vi "Read Data and Memory Array.vi"(7 "Channel (1)":i32=1, 8 "error in (no error)":errorcluster, 9 "Correction (0: Data)":u16(ring) items=["Formatted", "Corrected"], 10 "Source (0: Data)":u16(ring) items=["Data", "Memory"], 11 "VISA resource name":refnum<visa-resource-name>) -> (0 "error out":errorcluster, 1 "Secondary / Imaginary":dbl[](array[numeric]), 2 "Primary / Real":dbl[](array[numeric]), 3 "VISA resource name out":refnum<visa-resource-name>)   [LabVIEW 2011, in "Agilent ENA Series.lvlib"]
doc: "For the active trace of selected channel, reads out the formated or corrected data or memory array."
uses:
  Agilent ENA Series.lvlib
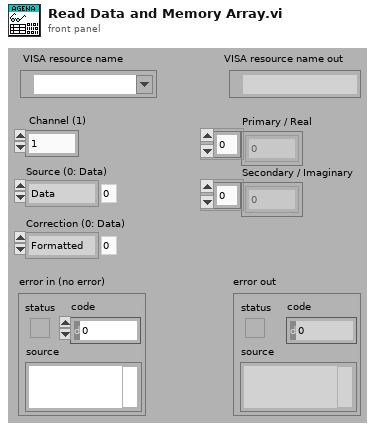
[diagram p1: front panel]
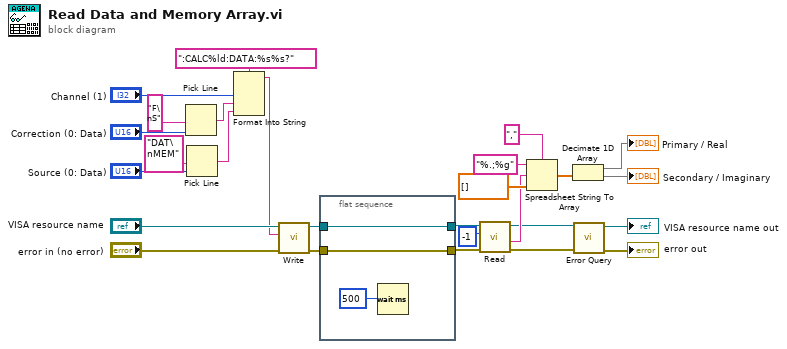
[diagram p0: block diagram]
diagram:
  n1 = Pick Line(multi-line string="F\nS", line index="Correction (0: Data)") -> (output string=w17:string)  [unwired: 1 in]
  n2 = Pick Line(multi-line string="DAT\nMEM", line index="Source (0: Data)") -> (output string=w14:string)  [unwired: 1 in]
  n3 = Format Into String(format string=":CALC%ld:DATA:%s%s?", "Channel (1)", w17, w14) -> (resulting string=w23:string)  [unwired: 2 in, 1 out]
  n4 = call "Write.vi"("error in (no error)"="error in (no error)", "String ()"=w23, "VISA resource name"="VISA resource name") -> ("error out"=w6:errorcluster, "VISA resource name out"=w8:refnum<visa-resource-name>)  [unwired: 6 in, 1 out]
  n5 = flat-sequence {
    tunnel: w8 -> [w30]
    tunnel: [w30] -> w7
    tunnel: w6 -> [w29]
    tunnel: [w29] -> w5
    frame #0 {
      n6 = Wait (ms)(milliseconds to wait=500) -> ()  [unwired: 1 out]
    }
  }
  n7 = call "Read.vi"("error in (no error)"=w5, "Number Of Bytes"=-1, "VISA resource name"=w7) -> ("error out"=w3:errorcluster, "String"=w13:string, "VISA resource name out"=w4:refnum<visa-resource-name>)  [unwired: 5 in, 1 out]
  n8 = Spreadsheet String To Array(delimiter (Tab)=",", format string="%.;%g", spreadsheet string=w13, array type (2D Dbl)=dbl[] []) -> (array=w11:dbl[])
  n9 = Decimate 1D Array(w11) -> (→"Primary / Real":dbl[], →"Secondary / Imaginary":dbl[])
  n10 = call "Error Query.vi"("error in (no error)"=w3, "VISA resource name"=w4) -> ("error out"=→"error out":errorcluster, "VISA resource name out"=→"VISA resource name out":refnum<visa-resource-name>)  [unwired: 6 in, 2 out]
